vi "Panel Averaging Values.vi"(0 "Default volume value":dbl, 11 "Error In":errorcluster) -> (4 "Scale Temp Coeff Out":dbl, 6 "Drum Volume":dbl=6.0, 8 "Out Strings":string[][](array[string]), 10 "MA Filter Size":i32=5, 15 "Error Out":errorcluster)   [LabVIEW 2012]
panel:
  in  "Help":bool
  in  "Drum Thermal Volume(>0)":string="13"
  in  "Scale Temp Coeff":string="0"
  in  "stop":bool
  in  "MA Filter Size(>0)":string="40"
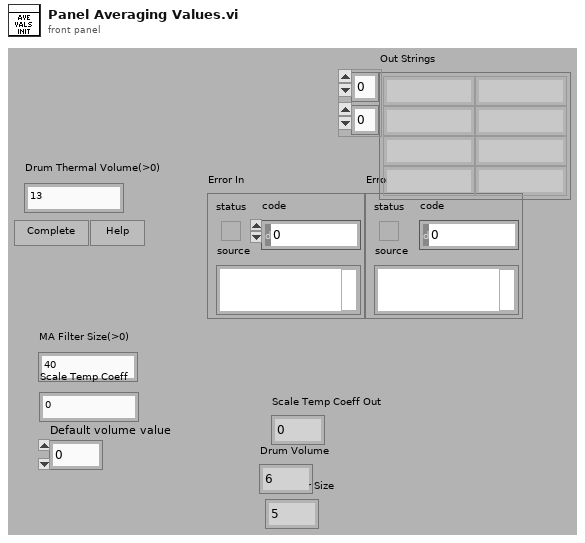
[diagram p1: front panel]
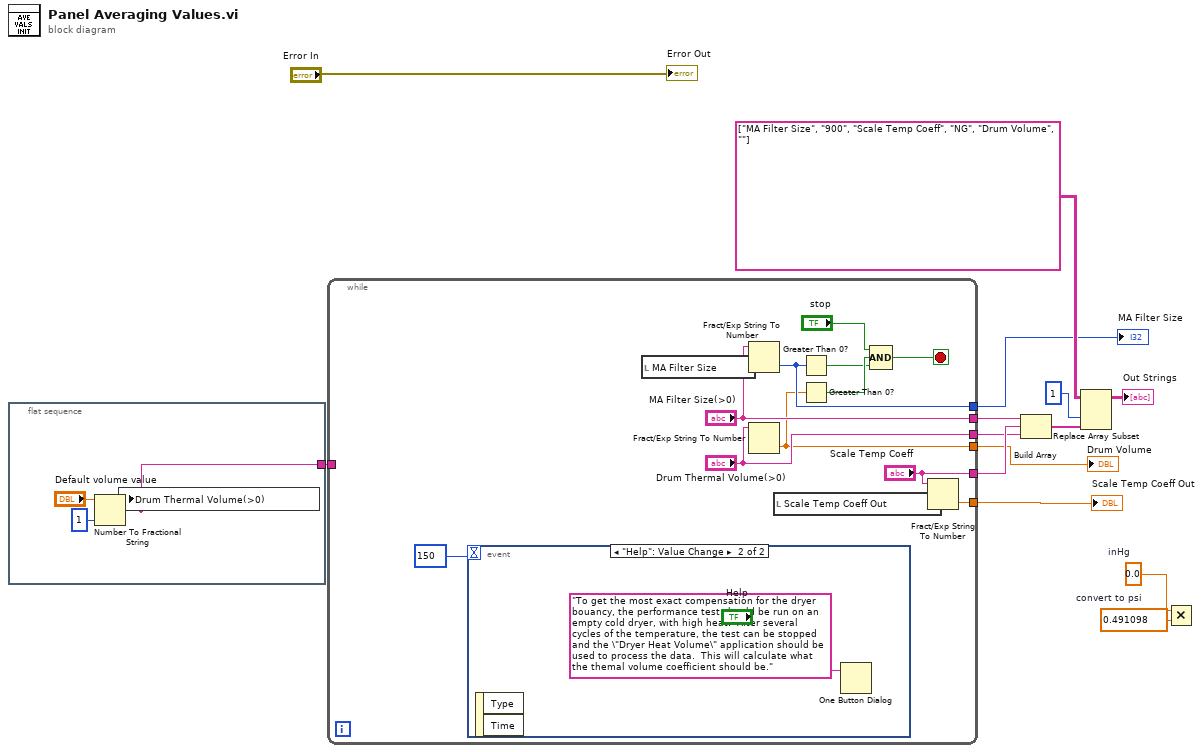
[diagram p0: block diagram]
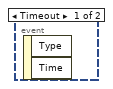
[diagram p2: hidden frame]
diagram:
  w8 = 0.0  # inHg
  w13 = 0.491098  # convert to psi
  n1 = flat-sequence {
    tunnel: [w15] -> w1
    frame #0 {
      n2 = Number To Fractional String(number="Default volume value", precision (6)=i16 1) -> (F-format string=w15:string)  [unwired: 2 in]
      n3 = local write "Drum Thermal Volume(>0)"(w15) -> ()
    }
  }
  n4 = while {
    tunnel: ["MA Filter Size(>0)"] -> w10
    tunnel: ["Scale Temp Coeff"] -> w7
    tunnel: ["Drum Thermal Volume(>0)"] -> w6
    tunnel: [w22] -> w4
    tunnel: [w20] -> w3
    tunnel: [w19] -> w2
    tunnel: w1 -> [_]
    stop <- w24 stop-if-true
    n5 = event shown="[1] \"Help\": Value Change" {
      selector: _ -> [_ _]
      dyn-events: _ -> [_ _]
      timeout: 150 ("milliseconds to wait") -> [_ _]
      event Timeout {
        n6 = event-data() -> ()  [unwired: 1 in, 2 out]
      }
      event "Help": Value Change {
        n7 = event-data() -> ()  [unwired: 1 in, 2 out]
        n8 = One Button Dialog(message="To get the most exact compensation for the dryer bouancy, the performance test should be run on an empty cold dryer, with high heat.  After several cycles of the temperature, the test can be stopped and the \"Dryer Heat Volume\" application should be used to process the data.  This will calculate what the themal volume coefficient should be.") -> ()  [unwired: 1 in, 1 out]
      }
    }
    n9 = local read "MA Filter Size"() -> (w23:i32)
    n10 = Fract/Exp String To Number(string="MA Filter Size(>0)", default (0 dbl)=w23) -> (number=w22:i32)  [unwired: 2 in, 1 out]
    n11 = Fract/Exp String To Number(string="Drum Thermal Volume(>0)") -> (number=w19:dbl)  [unwired: 3 in, 1 out]
    n12 = local read "Scale Temp Coeff Out"() -> (w21:dbl)
    n13 = Greater Than 0?(x=w22) -> (x > 0?=w25:bool)
    n14 = Greater Than 0?(x=w19) -> (x > 0?=w26:bool)
    n15 = Compound Arithmetic op=AND("stop", w26, w25) -> (w24:bool)
    n16 = Fract/Exp String To Number(string="Scale Temp Coeff", default (0 dbl)=w21) -> (number=w20:dbl)  [unwired: 2 in, 1 out]
  }
  "MA Filter Size" <- w4
  "Scale Temp Coeff Out" <- w3
  "Drum Volume" <- w2
  n17 = Build Array(w10, w7, w6) -> (w9:string[])
  n18 = Replace Array Subset(array=string[][] [["MA Filter Size", "900"], ["Scale Temp Coeff", "NG"], ["Drum Volume", ""]] ("appended array"), new element=w9, index (col)=1 ("disabled index (col)")) -> (→"Out Strings":string[][])  [unwired: 1 in]
  n19 = Multiply(x=w8, y=w13) -> ()  [unwired: 1 out]
  "Error Out" <- "Error In"
